vi "Log in-out.vi"(8 "error in (no error)":errorcluster {"code" format="%.0x"}, 9 "Input":enum16{"Log In", "Log Out"}(ring), 10 "Device Number (1)":i32=1, 11 "VISA Resource Name":refnum<visa-resource-name>) -> (0 "error out":errorcluster {"code" format="%.0x"}, 2 "Result":string, 3 "VISA Resource Name Out":refnum<visa-resource-name>)   [LabVIEW 2020]
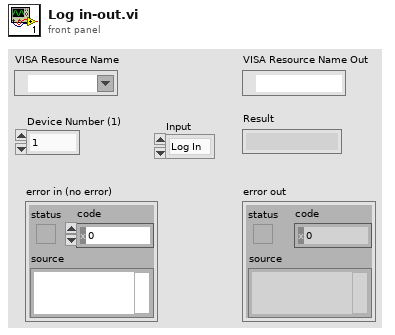
[diagram p1: front panel]
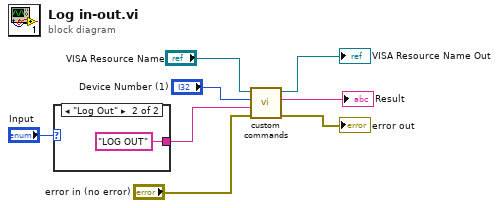
[diagram p0: block diagram]
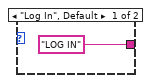
[diagram p2: hidden frame]
diagram:
  n1 = case shown="\"Log Out\"" "Input" {
    tunnel: ["LOG IN" ("format string") "LOG OUT" ("format string")] -> w1
    frame "Log In", Default {
    }
    frame "Log Out" {
    }
  }
  n2 = call "custom commands.vi"("error in (no error)"="error in (no error)", "format string"=w1, "Device Number (1)"="Device Number (1)", "VISA Resource Name"="VISA Resource Name") -> ("error out"=→"error out":errorcluster, "Result"=→"Result":string, "VISA Resource Name Out"=→"VISA Resource Name Out":refnum<visa-resource-name>)  [unwired: 5 in]
